vi "Arm2Execute_CtrlOnly.vi"(8 "ReverseLimitSwitch":bool, 9 "ForwardLimitSwitch":bool, 10 "SensorVel Deg/Sec":dbl, 11 "SensorPos Deg":dbl) -> (0 "Gravity Comp Output":dbl, 1 "OnTarget":bool, 2 "Arm Demand Deg":dbl, 3 "Motor Output":dbl)   [LabVIEW 2023]
doc: "Arm Execute for 2024 robot"
uses:
  <vilib>/Rock Robotics/WPI/ThirdParty/JAS_Junk/TrajLib/VI/numCmd_ObtainQueue_OneDbl.vi
  <vilib>/Rock Robotics/WPI/ThirdParty/JAS_Junk/TrajLib/Trajectory_Library.lvlib
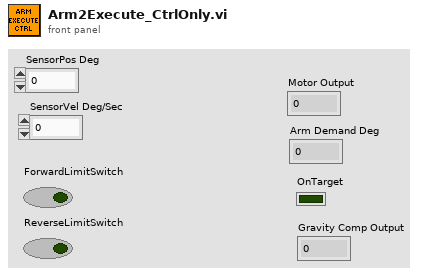
[diagram p1: front panel]
types:
  T1 = typedef "Trajectory_Library.lvlib/PosCtrl_Tuning_Type.ctl" = cluster{"Slope":dbl, "Offset":dbl, "Error Deadband":dbl, "At Reference Count":i32, "Negate Output":bool, "Max Allowd Position":dbl, "Min Allowd Position":dbl}
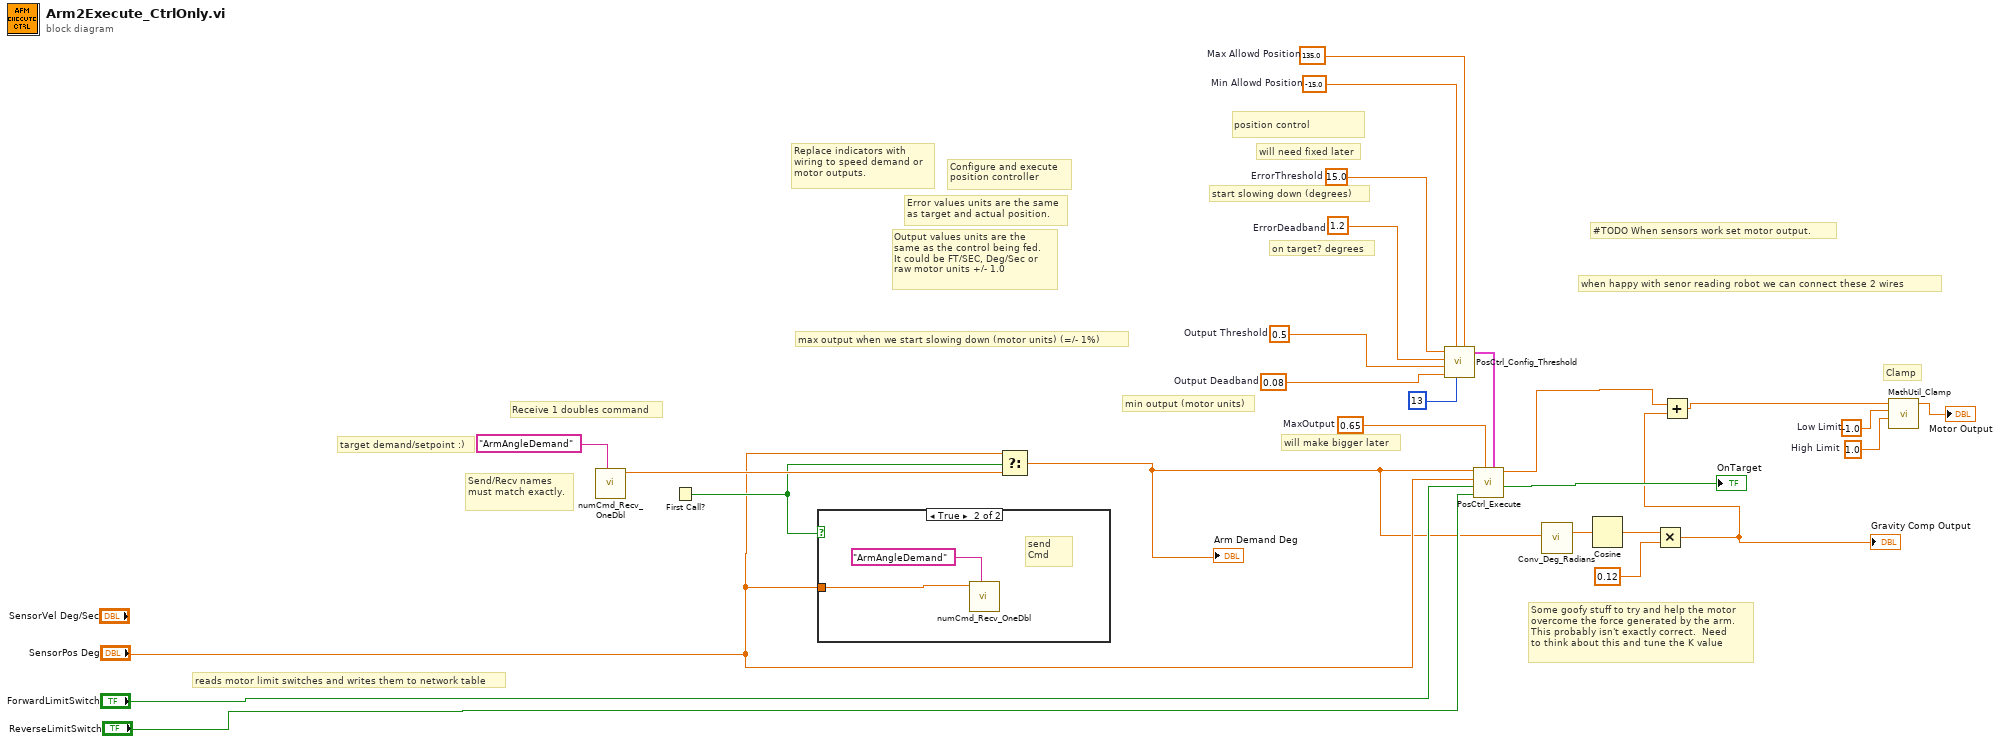
[diagram p0: block diagram]
diagram:
  w6 = 1.0  # High Limit
  w5 = -1.0  # Low Limit
  w12 = 135.0  # Max Allowd Position
  w13 = -15.0  # Min Allowd Position
  w26 = 0.65  # MaxOutput
  w24 = 15.0  # ErrorThreshold
  w23 = 1.2  # ErrorDeadband
  w22 = 0.5  # Output Threshold
  w21 = 0.08  # Output Deadband
  # "Some goofy stuff to try and help the motor\novercome the force generated by the arm.\nThis probably isn't exactly correct.  Need\nto think about this and tune the K value"
  # "Clamp"
  # "#TODO When sensors work set motor output."
  # "when happy with senor reading robot we can connect these 2 wires"
  # "min output (motor units)"
  # "max output when we start slowing down (motor units) (=/- 1%)"
  # "on target? degrees"
  # "start slowing down (degrees)"
  # "will make bigger later"
  # "target demand/setpoint :)"
  # "Send/Recv names\nmust match exactly."
  # "Receive 1 doubles command"
  # "position control"
  # "will need fixed later"
  # "reads motor limit switches and writes them to network table"
  # "Replace indicators with\nwiring to speed demand or\nmotor outputs."
  # "Output values units are the\nsame as the control being fed.  \nIt could be FT/SEC, Deg/Sec or\nraw motor units +/- 1.0"
  # "Error values units are the same \nas target and actual position."
  # "Configure and execute \nposition controller"
  n1 = call <vilib>:"numCmd_Recv_OneDbl.vi"("Command Name"="ArmAngleDemand") -> ("Value"=w19:dbl)  [unwired: 8 in, 2 out]
  n2 = First Call?() -> (First Call?: T/F=w18:bool)
  n3 = case shown="True" w18 {
    tunnel: "SensorPos Deg" -> [_ w27]
    frame False {
    }
    frame True {
      # "send\nCmd"
      n4 = call <vilib>:"numCmd_Recv_OneDbl.vi"("Command Name"="ArmAngleDemand", "Initial Value"=w27) -> ()  [unwired: 7 in, 3 out]
    }
  }
  n5 = Select(t="SensorPos Deg", s=w18, f=w19) -> (s? t:f=w2:dbl)
  "Arm Demand Deg" <- w2
  n6 = call <vilib>:"PosCtrl_Config_Threshold.vi"("Max Allowd Position"=w12, "At Reference Count"=13, "Min Allowd Position"=w13, "Output Deadband"=w21, "Output Threshold"=w22, "ErrorDeadband"=w23, "ErrorThreshold"=w24) -> ("PosCtrl_Config_Params"=w25:T1)  [unwired: 4 in]
  n7 = call <vilib>:"PosCtrl_Execute.vi"("PosCtrl_Config_Params"=w25, "MaxOutput"=w26, "Rev Limit Switch"="ReverseLimitSwitch", "Fwd Limit Switch"="ForwardLimitSwitch", "CurrentPosition"="SensorPos Deg", "TargetPosition"=w2) -> ("OnTarget"=→"OnTarget":bool, "Output"=w11:dbl)  [unwired: 3 in, 1 out]
  n8 = call <vilib>:"Conv_Deg_Radians.vi"("Degress"=w2) -> ("Radians"=w10:dbl)  [unwired: 10 in]
  n9 = Cosine(x=w10) -> (cos(x)=w9:dbl)
  n10 = Multiply(x=w9, y=0.12) -> (x*y=w1:dbl)
  "Gravity Comp Output" <- w1
  n11 = Add(x=w11, y=w1) -> (x+y=w4:dbl)
  n12 = call <vilib>:"MathUtil_Clamp.vi"("High Limit"=w6, "Low Limit"=w5, "Value"=w4) -> ("Result"=→"Motor Output":dbl)  [unwired: 8 in]
